vi "PythonNode_RemoveNoiseFromSignalUsingAnaconda.vi"() -> ()   [LabVIEW 2023]
doc: "This example demonstrates how to call a Python function in an Anaconda virtual environment. It uses python functions to create a signal, add noise to the signal and remove noise from the signal using fourier transform."
uses:
  <vilib>/Python/Open Anaconda Python Session.vi
panel:
  in  "Python version 2":string
  in  "Python version":string
  in  "Env name 2":string
  in  "Env name":string
  out "Sine wave with noise":cluster{dbl[], dbl[]}(graph)
  out "FFT noise removed":cluster{dbl[], dbl[]}(graph)
  out "FFT with noise":cluster{dbl[], dbl[]}(graph)
  out "Sine wave":cluster{dbl[], dbl[]}(graph)
  out "Retrieved signal after noise removal":cluster{dbl[], dbl[]}(graph)
  out "error out":errorcluster
  # "Overview: Demonstrates how to call a Python function in an Anaconda virtual environment and use packages installed inside the environment in the python code\nRequirements: \nAnaconda installed with the same bitness as LabVIEW.  The created anaconda environments should have numpy and scipy installed before running this VI. \nInstructions:\n1. Create two anaconda virtual environments and provide the names of the environments in the Env name and Env name 2 terminals. If you plan to use the same virtual environment you can give the same name in both of these terminals.\n2. Set the Python version and Python version 2 terminals to the versions in which the anaconda environments were created.\n3. Run the VI. You should see the results in the graphs.\n4. See comments on the block diagram of this VI for more information about how the call python node passes arguments and handles return values."
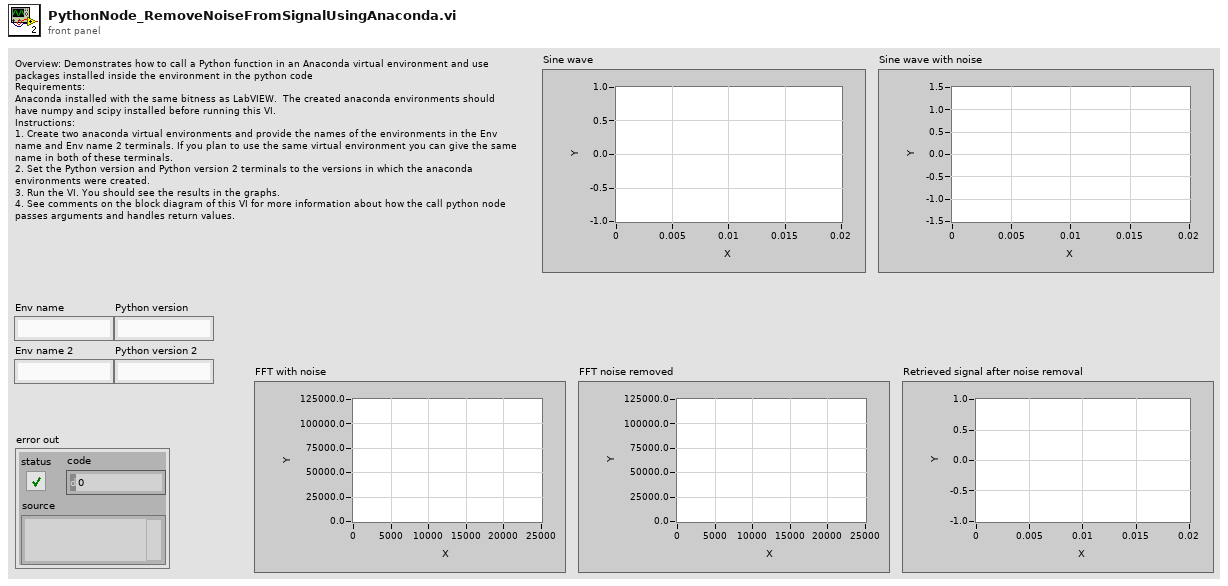
[diagram p1: front panel]
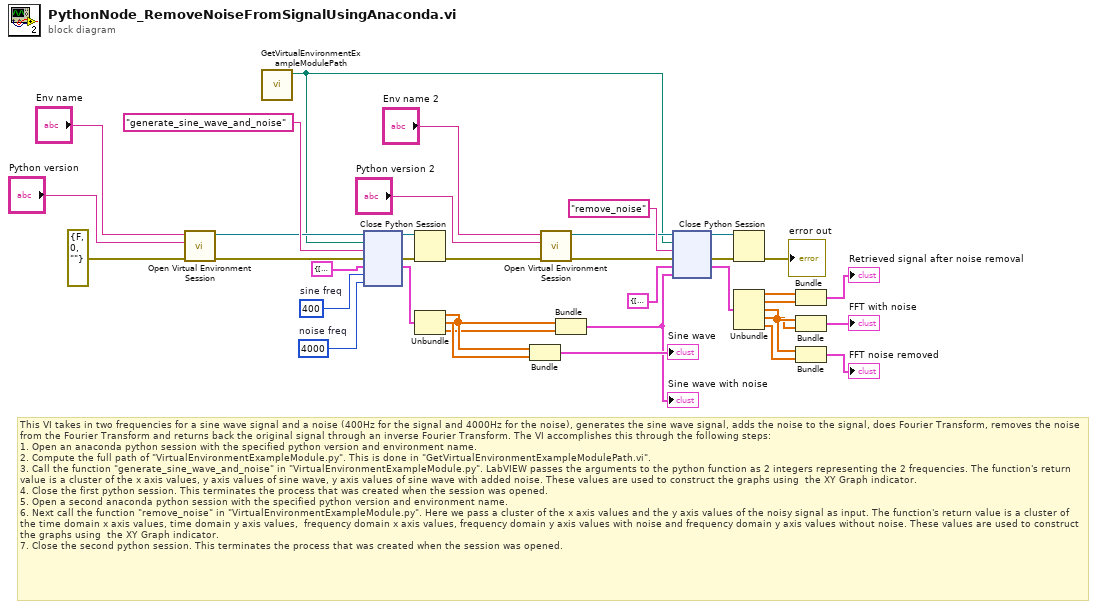
[diagram p0: block diagram]
diagram:
  w15 = 4000  # noise freq
  w33 = 400  # sine freq
  # "This VI takes in two frequencies for a sine wave signal and a noise (400Hz for the signal and 4000Hz for the noise), generates the sine wave signal, adds the noise to the signal, does Fourier Transform, removes the noise from the Fourier Transform and returns back the original signal through an inverse Fourier Transform. The VI accomplishes this through the following steps:\n1. Open an anaconda python session with the specified python version and environment name.\n2. Compute the full path of \"VirtualEnvironmentExampleModule.py\". This is done in \"GetVirtualEnvironmentExampleModulePath.vi\".\n3. Call the function \"generate_sine_wave_and_noise\" in \"VirtualEnvironmentExampleModule.py\". LabVIEW passes the arguments to the python function as 2 integers representing the 2 frequencies. The function's return value is a cluster of the x axis values, y axis values of sine wave, y axis values of sine wave with added noise. These values are used to construct the graphs using  the XY Graph indicator.\n4. Close the first python session. This terminates the process that was created when the session was opened.\n5. Open a second anaconda python session with the specified python version and environment name.\n6. Next call the function \"remove_noise\" in \"VirtualEnvironmentExampleModule.py\". Here we pass a cluster of the x axis values and the y axis values of the noisy signal as input. The function's return value is a cluster of the time domain x axis values, time domain y axis values,  frequency domain x axis values, frequency domain y axis values with noise and frequency domain y axis values without noise. These values are used to construct the graphs using  the XY Graph indicator.\n7. Close the second python session. This terminates the process that was created when the session was opened."
  n1 = call-poly <vilib>:"Open Virtual Environment Session.vi"("error in (no error)"=errorcluster {"status"=FALSE, "code"=0, "source"=""}, "Python version"="Python version", "Env name"="Env name") -> ("error out"=w10:errorcluster, "session out"=w13:refnum<k35>)  [unwired: 7 in]
  n2 = call "GetVirtualEnvironmentExampleModulePath.vi"() -> ("module path"=w3:path)  [unwired: 11 in]
  n3 = node(w13, w3, "generate_sine_wave_and_noise" ("function name"), w10, cluster{dbl[], dbl[], dbl[]} {[], [], []}, w33, w15) -> (w36:refnum<k35>, w37:errorcluster, w27:cluster{dbl[], dbl[], dbl[]})  [unwired: 2 in, 2 out]
  n4 = Close Python Session(session in=w36, error in=w37) -> (11:w4:errorcluster)
  n5 = Unbundle(w27) -> (w14:dbl[], w16:dbl[], w2:dbl[])
  n6 = Bundle(w14, w16) -> (→"Sine wave":cluster{dbl[], dbl[]})  [unwired: 1 in]
  n7 = call-poly <vilib>:"Open Virtual Environment Session.vi"("error in (no error)"=w4, "Python version"="Python version 2", "Env name"="Env name 2") -> ("error out"=w11:errorcluster, "session out"=w12:refnum<k35>)  [unwired: 7 in]
  n8 = Bundle(w14, w2) -> (w1:cluster{dbl[], dbl[]})  [unwired: 1 in]
  "Sine wave with noise" <- w1
  n9 = node(w12, w3, "remove_noise" ("function name"), w11, cluster{dbl[], dbl[], dbl[], dbl[], dbl[]} {[], [], [], [], []}, w1) -> (w30:refnum<k35>, w31:errorcluster, w25:cluster{dbl[], dbl[], dbl[], dbl[], dbl[]})  [unwired: 1 in, 2 out]
  n10 = Close Python Session(session in=w30, error in=w31) -> (11:→"error out":errorcluster)
  n11 = Unbundle(w25) -> (w24:dbl[], w23:dbl[], w21:dbl[], w20:dbl[], w19:dbl[])
  n12 = Bundle(w24, w23) -> (→"Retrieved signal after noise removal":cluster{dbl[], dbl[]})  [unwired: 1 in]
  n13 = Bundle(w21, w20) -> (→"FFT with noise":cluster{dbl[], dbl[]})  [unwired: 1 in]
  n14 = Bundle(w21, w19) -> (→"FFT noise removed":cluster{dbl[], dbl[]})  [unwired: 1 in]
